vi "getAll.vi"(8 "error in (no error)":errorcluster, 11 "instrument.PPMS3 in":refnum<class "instrument.PPMS3.lvclass">) -> (0 "error out":errorcluster, 2 "getAll":variant, 3 "instrument.PPMS out":refnum<class "instrument.PPMS3.lvclass">)   [LabVIEW 2019, in "instrument.PPMS3.lvclass"]
uses:
  instrument.PPMS3.lvclass
  C:/Users/patrick/Documents/GitHub/PPMS-Monitor-and-Control/lvsrc/instrument.PPMS/instrument.PPMS.lvclass
  instrument.PPMS/Typedefs/PPMS.getAll--cluster.ctl
  instrument.PPMS/instrument.PPMS.lvclass
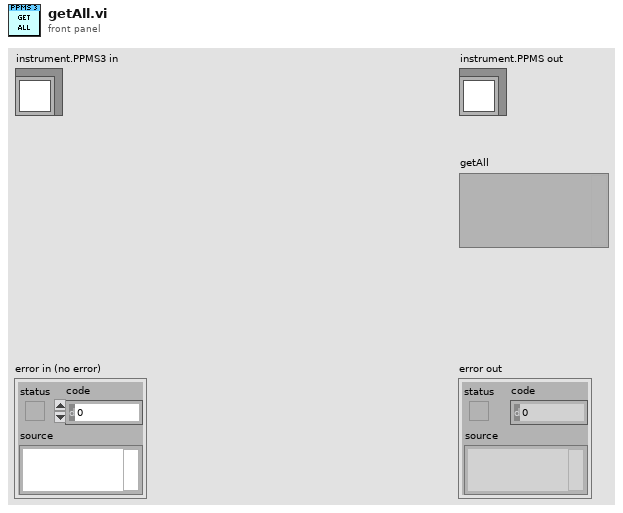
[diagram p1: front panel]
types:
  T1 = typedef "instrument.PPMS.lvclass/PPMS.getAll--cluster.ctl" = cluster{"Helium Level (%)":dbl, "Temperature (K)":dbl, "Temperature Status":string, "Magnetic Field (T)":dbl, "Magnet Status":string, "Position (°)":dbl}
  T2 = typedef "instrument.PPMS.lvclass/PPMS.Temperature Status--cluster.ctl" = cluster{"Temperature (K)":dbl, "Temperature Status":string}
  T3 = typedef "instrument.PPMS.lvclass/PPMS.Magnet Status--cluster.ctl" = cluster{"Field (T)":dbl, "Magnet Status":string}
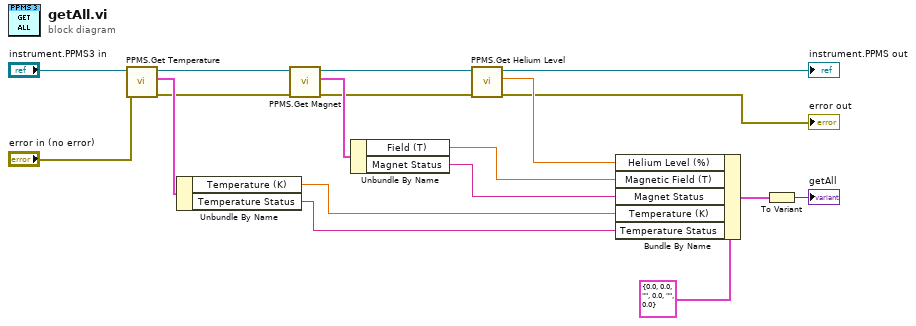
[diagram p0: block diagram]
diagram:
  n1 = call "PPMS.Get Temperature.vi"("error in (no error)"="error in (no error)", "instrument.PPMS"="instrument.PPMS3 in") -> ("error out"=w6:errorcluster, "Temperature Status"=w11:T2, "instrument.PPMS out"=w14:refnum<class "instrument.PPMS3.lvclass">)  [unwired: 7 in]
  n2 = Unbundle By Name(w11) -> ("Temperature (K)"=w10:dbl, "Temperature Status"=w9:string)
  n3 = call "PPMS.Get Magnet.vi"("error in (no error)"=w6, "instrument.PPMS"=w14) -> ("error out"=w5:errorcluster, "Magnet Status"=w8:T3, "instrument.PPMS out"=w13:refnum<class "instrument.PPMS3.lvclass">)  [unwired: 7 in]
  n4 = Unbundle By Name(w8) -> ("Field (T)"=w2:dbl, "Magnet Status"=w3:string)
  n5 = call "PPMS.Get Helium Level.vi"("error in (no error)"=w5, "instrument.PPMS"=w13) -> ("error out"=→"error out":errorcluster, "Helium Level (%)"=w16:dbl, "instrument.PPMS out"=→"instrument.PPMS out":refnum<class "instrument.PPMS3.lvclass">)  [unwired: 7 in]
  n6 = Bundle By Name(cluster=T1 {"Helium Level (%)"=0.0, "Temperature (K)"=0.0, "Temperature Status"="", "Magnetic Field (T)"=0.0, "Magnet Status"="", "Position (°)"=0.0} ("getAll"), "Helium Level (%)"=w16, "Magnetic Field (T)"=w2, "Magnet Status"=w3, "Temperature (K)"=w10, "Temperature Status"=w9) -> (w17:T1)
  n7 = To Variant(anything=w17) -> (Variant=→"getAll":variant)
